vi "Handle Debug Data.vi"(8 "error in (no error)":errorcluster, 10 "Debug Data.lvclass":refnum<class "Debug Data.lvclass">, 11 "Debug Data Event In":refnum<class "Debugger.lvclass">) -> (0 "error out":errorcluster, 3 "Debug Data Event Out":refnum<class "Debugger.lvclass">)   [LabVIEW 2020, in "Debugger.lvclass"]
uses:
  Debugger.lvclass
  C:/Users/anton/Documents/GitHub/triarc-debugger/source/Process/Debug Process.lvclass
  Debug Data/Debug Data.lvclass
  Process/Debug Process.lvclass/Debug Process.ctl
  <vilib>/Utility/error.llb/Clear Errors.vi
  <vilib>/Utility/error.llb/Error Cluster From Error Code.vi
  Process/Debug Process.lvclass
  State Analyzer/Debug State Analyzer.lvclass
  Debug Latest Message/Debug Latest Message.lvclass
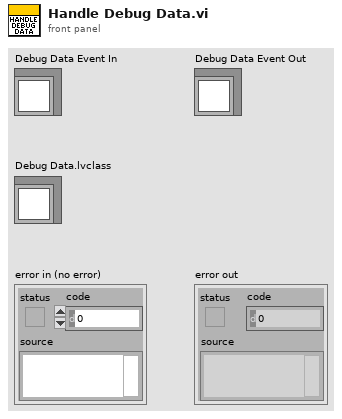
[diagram p1: front panel]
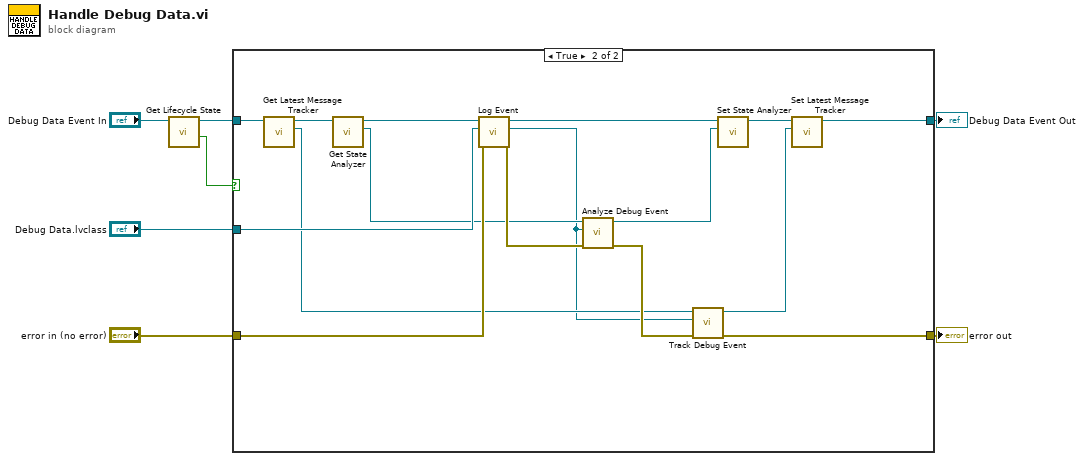
[diagram p0: block diagram]
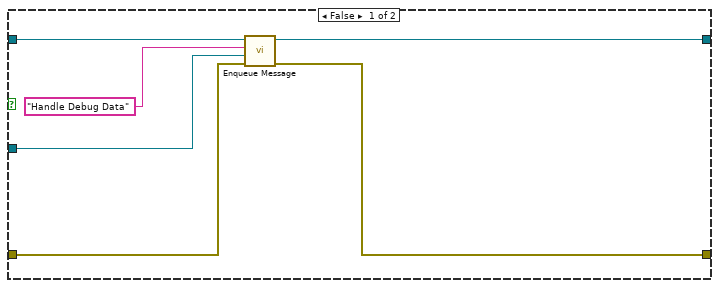
[diagram p2: hidden frame]
diagram:
  n1 = call "Get Lifecycle State.vi"("Process In"="Debug Data Event In") -> ("In Process Loop?"=w1:bool, "Process Out"=w2:refnum<class "Debugger.lvclass">)  [unwired: 7 in, 2 out]
  n2 = case shown="True" w1 {
    tunnel: [w13 w19] -> w6
    tunnel: "error in (no error)" -> [w12 w28]
    tunnel: [w11 w25] -> w4
    tunnel: "Debug Data.lvclass" -> [w10 w24]
    tunnel: w2 -> [w8 w29]
    frame False {
      n3 = call "Enqueue Message.vi"("error in (no error)"=w12, "Message Data"=w10, "Message"="Handle Debug Data", "Process In"=w8) -> ("error out"=w11:errorcluster, "Process Out"=w13:refnum<class "Debugger.lvclass">)  [unwired: 6 in]
    }
    frame True {
      n4 = call "Get Latest Message Tracker.vi"("Debugger in"=w29) -> ("Log"=w17:refnum<class "Debug Latest Message.lvclass">, "Debugger out"=w20:refnum<class "Debugger.lvclass">)  [unwired: 8 in, 1 out]
      n5 = call "Get State Analyzer.vi"("Debugger in"=w20) -> ("Log"=w21:refnum<class "Debug State Analyzer.lvclass">, "Debugger out"=w15:refnum<class "Debugger.lvclass">)  [unwired: 8 in, 1 out]
      n6 = call "Log Event.vi"("error in (no error)"=w28, "Debug Data.lvclass"=w24, "Debugger In"=w15) -> ("error out"=w27:errorcluster, "Debug Data out"=w16:refnum<class "Debug Data.lvclass">, "Debugger Out"=w14:refnum<class "Debugger.lvclass">)  [unwired: 6 in]
      n7 = call "Analyze Debug Event.vi"("error in (no error)"=w27, "Debug Data.lvclass"=w16, "Debug State Analyzer In"=w21) -> ("error out"=w26:errorcluster, "Debug State Analyzer Out"=w22:refnum<class "Debug State Analyzer.lvclass">)  [unwired: 7 in]
      n8 = call "Track Debug Event.vi"("error in (no error)"=w26, "Debug Data.lvclass"=w16, "Debug Latest Message In"=w17) -> ("error out"=w25:errorcluster, "Debug Latest Message Out"=w18:refnum<class "Debug Latest Message.lvclass">)  [unwired: 7 in]
      n9 = call "Set State Analyzer.vi"("Log"=w22, "Debugger in"=w14) -> ("Debugger out"=w23:refnum<class "Debugger.lvclass">)  [unwired: 8 in, 1 out]
      n10 = call "Set Latest Message Tracker.vi"("Log"=w18, "Debugger in"=w23) -> ("Debugger out"=w19:refnum<class "Debugger.lvclass">)  [unwired: 8 in, 1 out]
    }
  }
  "error out" <- w4
  "Debug Data Event Out" <- w6
